vi "SA Math - Scale Signals.vi"(0 "Signal IN":waveform(dbl)[](array[waveform]), 5 "error in (no error)":errorcluster, 6 "Anotate Signal Name":bool=TRUE, 7 "Scaling Factors":dbl[](array[numeric])=[1.0]) -> (14 "Signal OUT":waveform(dbl)[](array[waveform]), 19 "error out":errorcluster)   [LabVIEW 2022 SP3, in "GSwFormDSP.lvclass"]
uses:
  GSwFormDSP.lvclass
  Attribute List.ctl
  Attribute Options.ctl
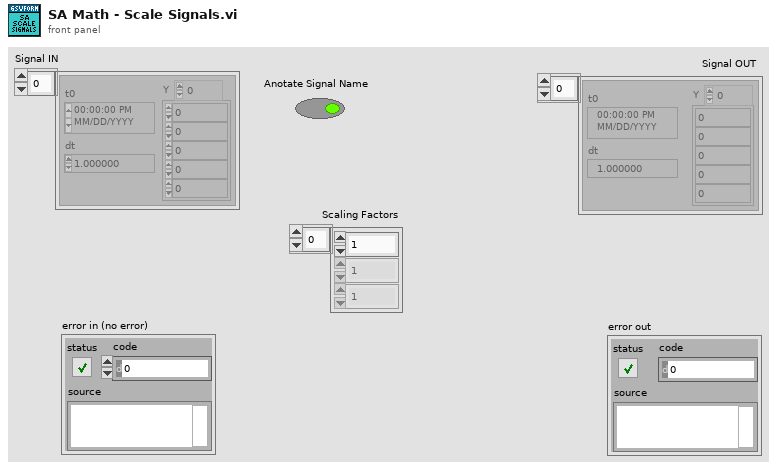
[diagram p1: front panel]
types:
  T1 = typedef "GSwFormDSP.lvclass/Attribute Options.ctl" = enum16{"Append to Attribute using \"( )\"", "Replace Attribute Value"}
  T2 = typedef "GSwFormDSP.lvclass/Attribute List.ctl" = string
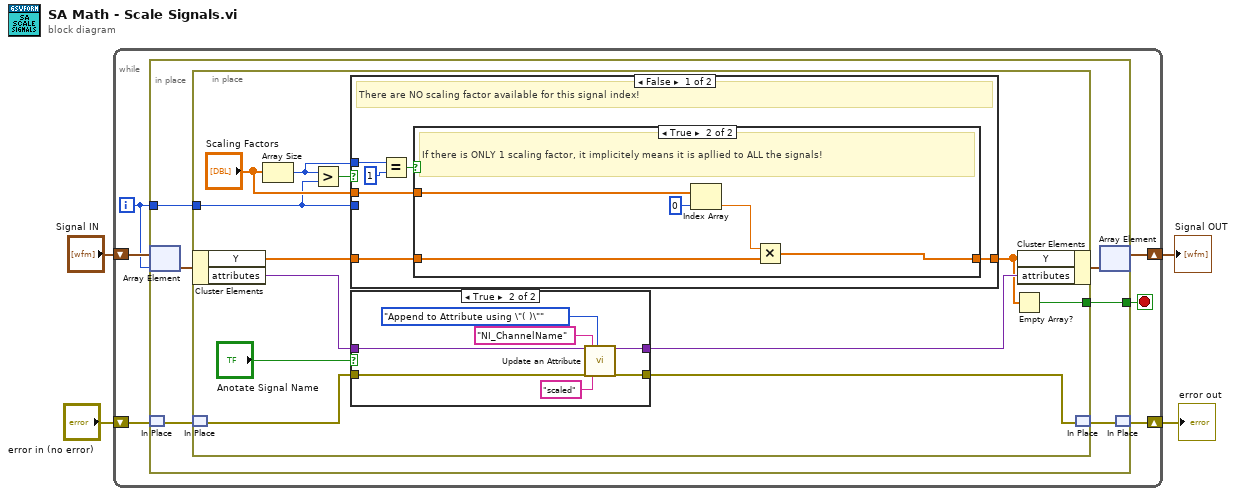
[diagram p0: block diagram]
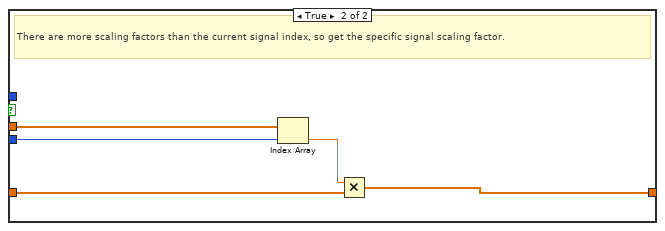
[diagram p3: hidden frame]
diagram:
  n1 = while {
    shift-right: [w9] -> w4
    shift-left: "Signal IN" -> [w10]
    shift-right: [w5] -> w1
    shift-left: "error in (no error)" -> [w6]
    i -> [w8]
    stop <- w7 stop-if-true
    n2 = in-place {
      in-place-border: w8 -> [w14]
      in-place-border: [w13] -> w7
      n3 = in-place-array #1(w10, w8) -> (w16:waveform(dbl))
      n4 = in-place-match #2(w6) -> (w12:errorcluster)
      n5 = in-place {
        in-place-border: w14 -> [w25]
        in-place-border: [w19] -> w13
        n6 = in-place-cluster #3(w16) -> ("Y"=w27:dbl[], "attributes"=w22:variant)
        n7 = in-place-match #4(w12) -> (w18:errorcluster)
        n8 = Array Size(array="Scaling Factors") -> (size(s)=w23:i32)
        n9 = Greater?(x=w23, y=w25) -> (0:w24:bool)
        n10 = case shown="False" w24 {
          tunnel: [w31 w45] -> w20
          tunnel: w27 -> [w30 w44]
          tunnel: "Scaling Factors" -> [w29 w42]
          tunnel: w25 -> [_ w43]
          tunnel: w23 -> [w34 _]
          frame False {
            # "There are NO scaling factor available for this signal index!"
            n11 = Equal?(x=w34, y=1 ("x")) -> (x = y?=w32:bool)
            n12 = case shown="True" w32 {
              tunnel: [w35 w38] -> w31
              tunnel: w30 -> [w35 w40]
              tunnel: w29 -> [_ w39]
              frame False {
                # "There are more than 1 scaling factors, but the signal index is greater than the number of available scaling factor, so implicetely it means to not do anything!"
              }
              frame True {
                # "If there is ONLY 1 scaling factor, it implicitely means it is apllied to ALL the signals!"
                n13 = Index Array(array=w39, index=0) -> (element=w37:dbl)
                n14 = Multiply(x=w37, y=w40) -> (x*y=w38:dbl[])
              }
            }
          }
          frame True {
            # "There are more scaling factors than the current signal index, so get the specific signal scaling factor."
            n15 = Index Array(array=w42, index=w43) -> (element=w41:dbl)
            n16 = Multiply(x=w41, y=w44) -> (x*y=w45:dbl[])
          }
        }
        n17 = case shown="True" "Anotate Signal Name" {
          tunnel: w22 -> [w47 w52]
          tunnel: [w47 w50] -> w21
          tunnel: w18 -> [w46 w49]
          tunnel: [w46 w48] -> w17
          frame False {
          }
          frame True {
            n18 = call "Update an Attribute.vi"("attributes in"=w52, "error in (no error)"=w49, "Attribute List"=T2 "NI_ChannelName", "Attribute Value"="scaled" ("string"), "Attribute Option"=Attribute_Options."Append to Attribute using \"( )\"") -> ("attributes out"=w50:variant, "error out"=w48:errorcluster)  [unwired: 13 in]
          }
        }
        n19 = Empty Array?(array=w20) -> (empty?=w19:bool)
        n20 = in-place-cluster #3("Y"=w20, "attributes"=w21) -> (w15:waveform(dbl))
        n21 = in-place-match #4(w17) -> (w11:errorcluster)
      }
      n22 = in-place-array #1(w15) -> (w9:waveform(dbl)[])  [unwired: 1 out]
      n23 = in-place-match #2(w11) -> (w5:errorcluster)
    }
  }
  "Signal OUT" <- w4
  "error out" <- w1
